vi "Add Output.vi"(0 "Output Terminal in":refnum<class "Output Terminal.lvclass">, 5 "Comiplation message":T1[](array[typedef]), 11 "error in (no error)":errorcluster) -> (4 "Output Terminal out":refnum<class "Output Terminal.lvclass">, 15 "error out":errorcluster)   [LabVIEW 2019, in "LSL.lvlib" / "Output Terminal.lvclass"]
uses:
  Output Terminal.lvclass
  common/function utils/Validate_message.ctl
  common/function utils/Validate_MessageStatus.ctl
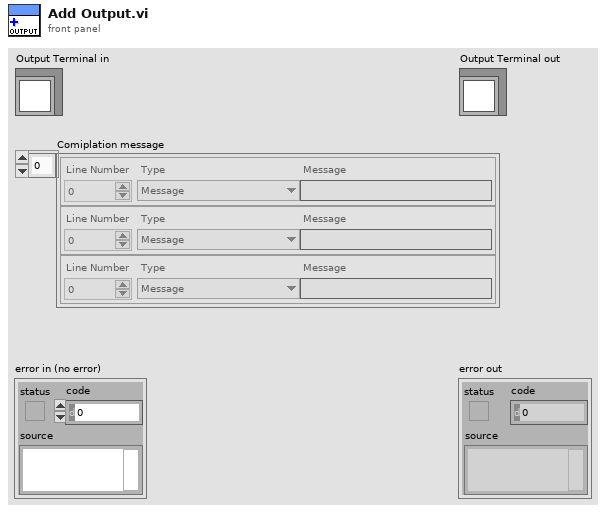
[diagram p1: front panel]
types:
  T1 = typedef "Validate_message.ctl" = cluster{"Line Number":i64, "Type":T2, "Message":string}
  T2 = typedef "Validate_MessageStatus.ctl" = enum16{"Message", "Warning", "Error"}
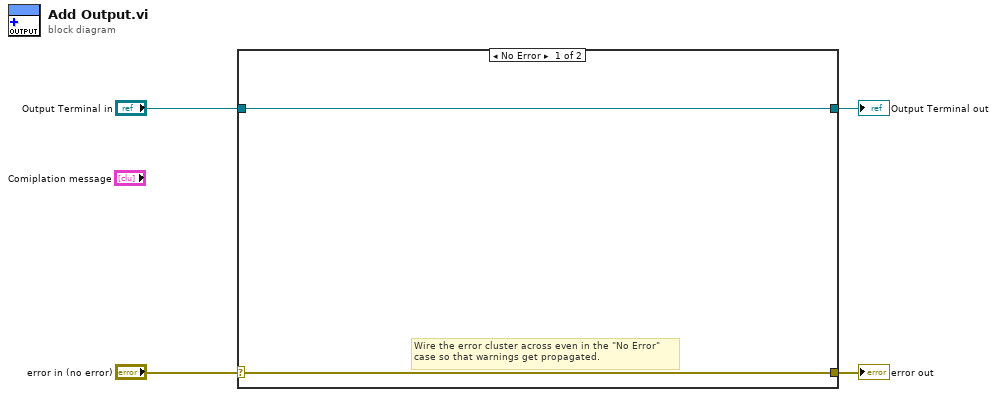
[diagram p0: block diagram]
diagram:
  n1 = case shown="No Error" "error in (no error)" {
    selector: "error in (no error)" -> [w5 w8]
    tunnel: [w5 w8] -> w3
    tunnel: [w6 w7] -> w1
    tunnel: "Output Terminal in" -> [w6 w7]
    frame No Error {
      # "Wire the error cluster across even in the \"No Error\"\ncase so that warnings get propagated."
    }
    frame Error {
    }
  }
  "error out" <- w3
  "Output Terminal out" <- w1
